vi "Publish.vi"(8 "error in (no error)":errorcluster, 10 "message":T1, 11 "service in":refnum<class "IcmMessageService.lvclass">) -> (0 "error out":errorcluster, 3 "service out":refnum<class "IcmMessageService.lvclass">)   [LabVIEW 2017, in "IcmMessageService.lvclass"]
doc: "Publishes a message to the message bus."
uses:
  <vilib>/addons/InsightCM/MessageBus/MessageService/IcmMessageService.lvclass
  <vilib>/addons/InsightCM/MessageBus/Base/controls/Message.ctl
  <vilib>/addons/InsightCM/MessageBus/Base/controls/MessageHeader.ctl
  <vilib>/addons/InsightCM/MessageBus/Base/controls/KeyValuePair.ctl
  <vilib>/addons/InsightCM/MessageBus/MessageService/IcmMessageService.lvclass/IcmMessageService.ctl
  C:/Program Files (x86)/National Instruments/LabVIEW 2017/vi.lib/addons/InsightCM/Binaries/LabviewMessageAdapter.dll
  Binaries/LabviewMessageAdapter.dll
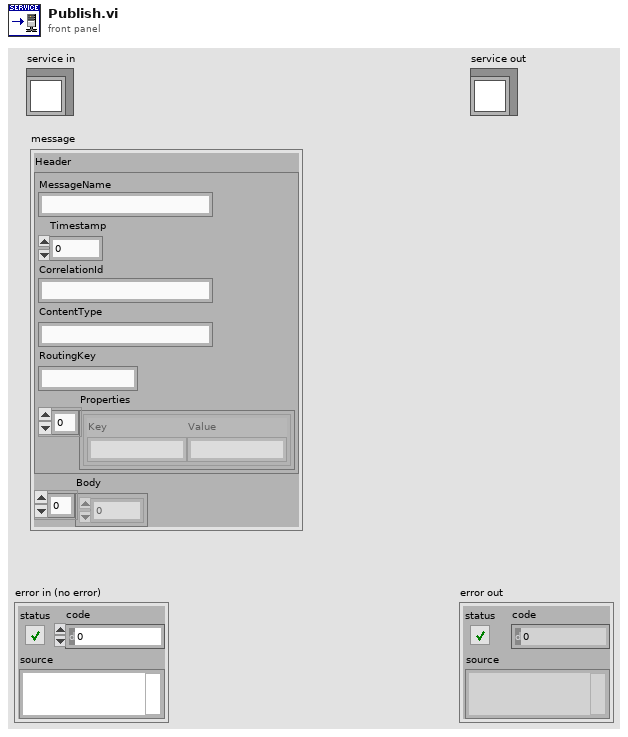
[diagram p1: front panel]
types:
  T1 = typedef "Message.ctl" = cluster{"Header":T2, "Body":u8[]}
  T2 = typedef "MessageHeader.ctl" = cluster{"MessageName":string, "Timestamp":i64, "CorrelationId":string, "ContentType":string, "RoutingKey":string, "Properties":T3[]}
  T3 = typedef "KeyValuePair.ctl" = cluster{"Key":string, "Value":string}
  T4 = typedef "MessageServiceDvr.ctl" = refnum<data-value>
  T5 = typedef "MessageServiceData.ctl" = cluster{"Service":refnum<k24>}
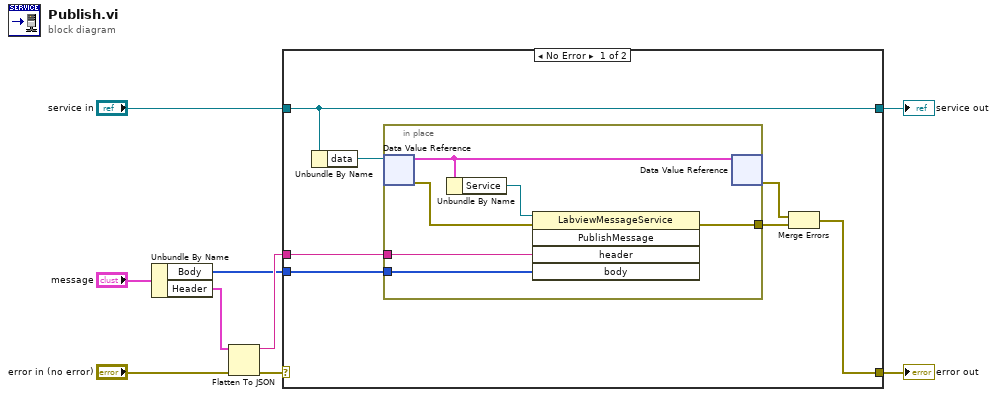
[diagram p0: block diagram]
diagram:
  n1 = Unbundle By Name("message") -> ("Body"=w1:u8[], "Header"=w2:T2)
  n2 = Flatten To JSON(anything=w2, error in (no error)="error in (no error)") -> (JSON string=w4:string, 11:w5:errorcluster)  [unwired: 1 in]
  n3 = case shown="No Error" w5 {
    selector: w5 -> [_ w24]
    tunnel: [w12 w24] -> w9
    tunnel: [w16 w23] -> w7
    tunnel: "service in" -> [w16 w23]
    tunnel: w4 -> [w11 _]
    tunnel: w1 -> [w10 _]
    frame No Error {
      n4 = Unbundle By Name(w16) -> ("data"=w15:T4)
      n5 = in-place {
        in-place-border: [w19] -> w13
        in-place-border: w11 -> [w18]
        in-place-border: w10 -> [w17]
        n6 = in-place-dvr #1(w15) -> (w22:T5, w20:errorcluster)
        n7 = Unbundle By Name(w22) -> ("Service"=w21:refnum<k24>)
        n8 = invoke class="LabviewMessageService" method="PublishMessage"(reference=w21, error in=w20, "header"=w18, "body"=w17) -> (error out=w19:errorcluster)  [unwired: 1 in, 4 out]
        n9 = in-place-dvr #1(w22) -> (w14:errorcluster)  [unwired: 1 out]
      }
      n10 = Merge Errors(w14, w13) -> (w12:errorcluster)
    }
    frame Error {
    }
  }
  "error out" <- w9
  "service out" <- w7
